vi "Lecroy_fast_wait&get_trace.vi"(1 "Activated channels":u16[](array[numeric]), 2 "stop (ref)":refnum<vi>, 3 "start (ref)":refnum<vi>, 4 "VISA resource name":refnum<visa-resource-name>) -> (0 "measures":dbl[][](array[numeric]))   [LabVIEW 2013]
uses:
  LeCroy Wave Series/LeCroy Wave Series.lvlib
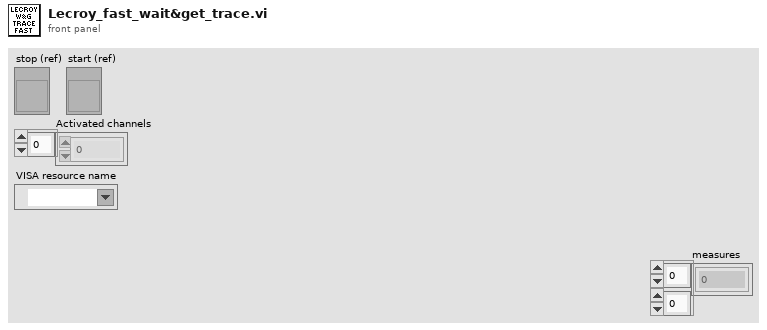
[diagram p1: front panel]
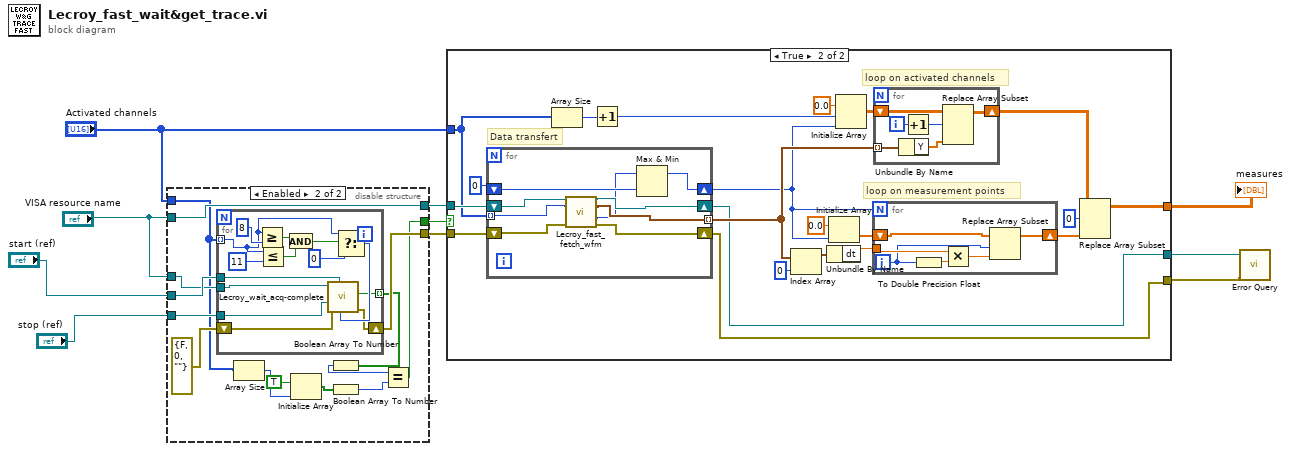
[diagram p0: block diagram]
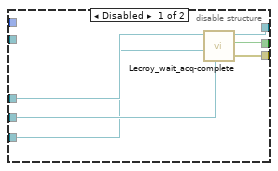
[diagram p2: hidden frame]
diagram:
  n1 = disable-structure shown="Enabled" {
    disable-tunnel: [w16 w21] -> w10
    disable-tunnel: [w15 w25] -> w9
    disable-tunnel: [w14 w27] -> w8
    disable-tunnel: "VISA resource name" -> [w13 w28]
    disable-tunnel: "start (ref)" -> [w12 w30]
    disable-tunnel: "stop (ref)" -> [w11 w29]
    disable-tunnel: "Activated channels" -> [_ w24]
    disable-tunnel: "VISA resource name" -> [_ w27]
    frame Disabled {
      n2 = call "Lecroy_wait_acq-complete.vi"("start (ref)"=w12, "stop (ref)"=w11, "VISA resource name"=w13) -> ("error out"=w15:errorcluster, "Complete"=w16:bool, "VISA resource name out"=w14:refnum<visa-resource-name>)  [unwired: 2 in, 4 out]
    }
    frame Enabled {
      n3 = for {
        tunnel: w24 -> [w39] mode=indexing
        tunnel: w30 -> [w37]
        tunnel: w29 -> [w36]
        tunnel: w28 -> [w35]
        tunnel: [w33] -> w17 mode=indexing
        shift-right: [w31] -> w25
        shift-left: errorcluster {"status"=FALSE, "code"=0, "source"=""} ("error out") -> [w32]
        n4 = Greater Or Equal?(x=w39, y=u16 8) -> (x >= y?=w42:bool)
        n5 = Less Or Equal?(x=w39, y=u16 11) -> (x <= y?=w41:bool)
        n6 = And(x=w42, y=w41) -> (x .and. y?=w40:bool)
        n7 = Select(t=w39, s=w40, f=u16 0) -> (s? t:f=w34:u16)
        n8 = call "Lecroy_wait_acq-complete.vi"("INR bit (0)"=w34, "start (ref)"=w37, "error in (no error)"=w32, "stop (ref)"=w36, "VISA resource name"=w35) -> ("error out"=w31:errorcluster, "Complete"=w33:bool)  [unwired: 1 in, 4 out]
      }
      n9 = Array Size(array=w24) -> (size(s)=w23:i32)
      n10 = Initialize Array(TRUE ("Complete"), w23) -> (w20:bool[])
      n11 = Boolean Array To Number(Boolean array=w17) -> (number=w18:u32)
      n12 = Boolean Array To Number(Boolean array=w20) -> (number=w19:u32)
      n13 = Equal?(x=w18, y=w19) -> (x = y?=w21:bool)
    }
  }
  n14 = case shown="True" w10 {
    tunnel: "Activated channels" -> [_ w63]
    tunnel: w8 -> [w46 w67]
    tunnel: w9 -> [w45 w66]
    tunnel: [_ w53] -> w7
    tunnel: [w46 w52] -> w6
    tunnel: [w45 w51] -> w5
    frame False {
    }
    frame True {
      # "Data transfert"
      # "loop on measurement points"
      # "loop on activated channels"
      n15 = for {
        tunnel: w63 -> [w83] mode=indexing
        shift-right: [w85] -> w51
        shift-left: w66 -> [w86]
        shift-right: [w82] -> w52
        shift-left: w67 -> [w84]
        shift-right: [w87] -> w48
        shift-left: u32 0 ("Number Of Data Points") -> [w88]
        tunnel: [w81] -> w57 mode=indexing
        n16 = call "Lecroy_fast_fetch_wfm.vi"("VISA resource name"=w84, "Source (0: Channel 1)"=w83, "error in (no error)"=w86) -> ("VISA resource name out"=w82:refnum<visa-resource-name>, "Waveform Graph"=w81:waveform(dbl), "Number Of Data Points"=w80:u32, "error out"=w85:errorcluster)  [unwired: 9 in]
        n17 = Max & Min(x=w80, y=w88) -> (max(x,y)=w87:u32)  [unwired: 1 out]
      }
      n18 = Array Size(array=w63) -> (size(s)=w50:i32)
      n19 = Increment(x=w50) -> (x+1=w47:i32)
      n20 = Index Array(array=w57, index=0 ("indice")) -> (element=w58:waveform(dbl))
      n21 = Unbundle By Name(w58) -> ("dt"=w56:dbl)
      n22 = Initialize Array(0.0 ("élément"), w48) -> (w62:dbl[])
      n23 = Initialize Array(0.0 ("élément"), w47, w48) -> (w60:dbl[][])
      n24 = for {
        N: w48 -> [_]
        tunnel: w56 -> [w73]
        shift-right: [w70] -> w54
        shift-left: w62 -> [w72]
        i -> [w68]
        n25 = To Double Precision Float(number=w68) -> (double precision float=w69:dbl)
        n26 = Multiply(x=w73, y=w69) -> (x*y=w71:dbl)
        n27 = Replace Array Subset(array=w72, new element=w71, index=w68) -> (w70:dbl[])
      }
      n28 = for {
        tunnel: w57 -> [w77] mode=indexing
        shift-right: [w75] -> w55
        shift-left: w60 -> [w79]
        i -> [w78]
        n29 = Unbundle By Name(w77) -> ("Y"=w76:dbl[])
        n30 = Increment(x=w78) -> (x+1=w74:i32)
        n31 = Replace Array Subset(array=w79, new element=w76, index (row)=w74) -> (w75:dbl[][])  [unwired: 1 in]
      }
      n32 = Replace Array Subset(array=w55, new element=w54, index (row)=0) -> (w53:dbl[][])  [unwired: 1 in]
    }
  }
  "measures" <- w7
  n33 = call "Error Query.vi"("error in (no error)"=w5, "VISA resource name"=w6) -> ()  [unwired: 10 out]
